vi "Query_source_settings_menu.vi"(8 "error in (no error)":errorcluster) -> (0 "error out":errorcluster, 1 "Cancelled?":bool, 3 "Output cluster":T1={"Integer Timestamp"=0, "Einzel Voltage"=0.0, "Needle Voltage"=0.0, "Frequency"=1.0, "Width (ms) : 0.1 "=0.05, "Desired Amplitude (V)"=0.0, "X Voltage"=0.0, "Y Voltage"=0.0, "Settings ID"="", "ID#"=0} {"Needle Voltage" min=0.0 max=10.0 step=0.01 format="%.2g"; "Y Voltage" min=0.0 max=9.0 step=0.01 format="%.2g"; "X Voltage" min=0.0 max=9.0 step=0.01 format="%.2g"; "Einzel Voltage" min=0.0 max=10.0 step=0.01 format="%.2g"; "Desired Amplitude (V)" min=0.0 max=10.0 step=0.01 format="%5.2f"; "Width (ms) : 0.1" min=0.05 max=5.0 step=0.01 format="%6.2f"; "Frequency" min=1.0 max=100.0 step=0.01 format="%.1f"})   [LabVIEW 2013]
doc: "Displays a standard dialog box that prompts users to enter information, such as a user name and password.\n--------------------\n\nThis Express VI is configured as follows:\n\nMessage to Display to the User:\nThe inputs are: \nNumber: Upper Timestamp Range\nNumber: Lower Timestamp Range\nNumber: Settings ID"
uses:
  Controls/dust_soruce_control.ctl
  Controls/Source_settings_select.ctl
  <vilib>/Utility/miscctls.llb/LVPointTypeDef.ctl
panel:
  out "Source Control Array":T1[](array[typedef]) {"Needle Voltage" min=0.0 max=10.0 step=0.01 format="%.2g"; "Y Voltage" min=0.0 max=9.0 step=0.01 format="%.2g"; "X Voltage" min=0.0 max=9.0 step=0.01 format="%.2g"; "Einzel Voltage" min=0.0 max=10.0 step=0.01 format="%.2g"; "Desired Amplitude (V)" min=0.0 max=10.0 step=0.01 format="%5.2f"; "Width (ms) : 0.1" min=0.05 max=5.0 step=0.01 format="%6.2f"; "Frequency" min=1.0 max=100.0 step=0.01 format="%.1f"}
  in  "Settings Type":T2
  in  "Clear Filter":bool
  in  "Tag Filter":T3
  in  "Load Settings":bool caption="OK2"
  in  "Cancel":bool
  in  "Settings ID":i32(ring) items=["Awesome settings that work"=30, "Awesome settings that work"=31, "Working settings"=35, "Working settings"=36, "Working settings"=37, "Working settings"=38, "Working settings"=39, ""=42, "Test"=43, "Test"=44, "Test"=46, "Test 1"=47, "Test 1"=48, "Anna's Settings"=49, "test of width"=51, "Anna's Settings (Updated with working Giraffes)"=72, "Anna's Settings (Updated with working Giraffes)"=73, "test"=75, "test"=76, "test 1"=77, "test 1"=78, "test 3"=82, "test 4"=83, "Anna's Settings"=86, "Anna's Settings1"=87, "test mctesty"=88, "test mctesty"=89, "Test\""=91, "Test\""=92, "this is a \"test\" setting"=93, "Test 'Test' \"Test\" test test."=97, "testsaved at  10/25/2012 3:26:30 PM"=101, "test (saved at  10/25/2012 3:26:53 PM)"=103, "Leela (saved at  11/2/2012 10:29:09 AM)"=112, "Light flash run 2 (saved at  11/13/2012 12:55:50 PM)"=184, "AnnaWorking (saved at  11/19/2012 12:04:04 PM)"=198, "AnnaWorking (saved at  11/19/2012 2:06:00 PM)"=200, "AnnaWorking (saved at  11/19/2012 4:00:30 PM)"=201, "DCS testing 1 (saved at  12/10/2012 3:10:12 PM)"=237, " (saved at  12/10/2012 6:22:18 PM)"=241, " (saved at  12/13/2012 1:54:08 PM)"=258, " (saved at  12/18/2012 1:57:42 PM)"=267, " (saved at  12/18/2012 1:57:45 PM)"=268, " (saved at  12/18/2012 1:58:11 PM)"=269, "fibera (saved at  12/18/2012 1:58:19 PM)"=270, "fibera (saved at  12/18/2012 1:58:37 PM)"=271, "fibera (saved at  12/18/2012 4:18:34 PM)"=272, "fibera (saved at  12/21/2012 11:52:02 AM)"=277, "Evan (saved at  2/11/2013 11:10:44 AM)"=346, "Evan (saved at  2/11/2013 11:10:45 AM)"=347, "Evan (saved at  2/11/2013 11:10:47 AM)"=348, "Evan (saved at  2/11/2013 11:10:48 AM)"=349, "Evan (saved at  2/11/2013 11:10:48 AM)"=350, "Evan (saved at  2/11/2013 11:10:48 AM)"=351, "Evan (saved at  2/11/2013 11:10:48 AM)"=352, "Evan (saved at  2/11/2013 11:10:48 AM)"=353, "Evan (saved at  2/11/2013 11:10:49 AM)"=354, "Evan (saved at  2/11/2013 11:10:50 AM)"=355, "Evan (saved at  2/11/2013 11:10:50 AM)"=356, "MINE (saved at  2/14/2013 11:07:05 AM)"=365, "MINE (saved at  2/14/2013 11:07:30 AM)"=366, "this (saved at  2/14/2013 12:24:07 PM)"=367, "this (saved at  2/14/2013 12:24:20 PM)"=368, "this (saved at  2/14/2013 12:24:20 PM)"=369, "this (saved at  2/14/2013 12:24:20 PM)"=370, "this (saved at  2/14/2013 12:24:21 PM)"=371, "this (saved at  2/14/2013 12:24:21 PM)"=372, "this (saved at  2/14/2013 12:24:21 PM)"=373, "MINE (saved at  2/14/2013 3:45:56 PM)"=374, " (saved at  2/18/2013 2:58:35 PM)"=379, "Evan (saved at  2/18/2013 2:58:43 PM)"=380, " (saved at  2/18/2013 5:00:50 PM)"=389, " (saved at  2/19/2013 11:55:54 AM)"=391, "Evan (saved at  2/19/2013 11:56:13 AM)"=392, "YABBADABBADOO (saved at  3/1/2013 10:24:08 AM)"=415, "Best Settings (saved at  5/6/2013 4:16:23 PM)"=473, "Aiming (saved at  5/21/2013 11:06:06 AM)"=548, "EVAN USE THESE SETTINGS (Freq: 15-20 ish) (saved at  5/21/2013 3:57:32 PM)"=552, "EVAN USE THESE SETTINGS (Freq: 15-20 ish) (saved at  5/21/2013 3:57:43 PM)"=553, "stereo (saved at  5/28/2013 12:22:49 PM)"=567, "stereo (saved at  5/28/2013 12:23:26 PM)"=568, "stereo (saved at  5/28/2013 1:04:18 PM)"=569, "stereo (saved at  5/28/2013 1:33:34 PM)"=570, "stereo (saved at  5/28/2013 1:33:38 PM)"=571, "test (saved at  5/31/2013 9:30:39 AM)"=573, "stereo (saved at  6/5/2013 4:20:29 PM)"=585, "stereo (saved at  6/11/2013 11:18:15 AM)"=590, "stereo (saved at  6/18/2013 5:04:42 PM)"=596, "stereo (saved at  6/20/2013 2:33:58 PM)"=600, "stereo (saved at  6/28/2013 10:16:59 AM)"=607, "stereo (saved at  7/16/2013 1:47:31 PM)"=611, "stereo (saved at  8/20/2013 5:15:00 PM)"=630, "stereo high (saved at  8/21/2013 11:26:34 AM)"=632, "stereo high (saved at  8/21/2013 2:57:56 PM)"=634, "stereo high focus better? (saved at  8/21/2013 4:20:43 PM)"=635, "stereo high focus better? (saved at  8/21/2013 4:22:36 PM)"=636, "aiming (saved at  8/27/2013 9:46:16 AM)"=640, "eric initial highspeed (saved at  8/29/2013 9:32:19 AM)"=641, "eric highspeed (saved at  8/29/2013 10:11:17 AM)"=642, "eric high S1 (saved at  8/29/2013 12:56:28 PM)"=643, "eric  S3 (saved at  8/29/2013 1:27:03 PM)"=645, "Solar Cell (saved at  9/17/2013 11:09:09 AM)"=656, "Solar Cell (saved at  9/17/2013 1:21:46 PM)"=657, "trytomakeolivineGO (saved at  9/23/2013 2:27:29 PM)"=664, "trytomakeolivineGO (saved at  9/23/2013 2:46:08 PM)"=666, "trytomakeolivineGO (saved at  9/23/2013 3:18:03 PM)"=667, "trytomakeolivineGO (saved at  9/23/2013 5:08:18 PM)"=669, "trytomakeolivineGO (saved at  9/24/2013 9:55:57 AM)"=673, "olivinehigh (saved at  9/24/2013 5:17:27 PM)"=679, "olivineisshooting (saved at  9/25/2013 10:27:24 AM)"=682, "olivineisshooting (saved at  9/25/2013 10:28:24 AM)"=683, "olivineisshooting? (saved at  9/25/2013 2:02:32 PM)"=684, "reallyhigh (saved at  9/26/2013 2:34:23 PM)"=690, "OLIVINE (saved at  9/30/2013 9:57:31 AM)"=693, "OLIVINE (saved at  9/30/2013 11:18:54 AM)"=694, "OLIVINE (saved at  9/30/2013 5:13:02 PM)"=696, "OLIVINE (saved at  10/2/2013 10:01:39 AM)"=699, "OLIVINE (saved at  10/2/2013 2:01:51 PM)"=701, "OLIVINE 1MV (saved at  10/2/2013 3:00:49 PM)"=703, "OLIVINE (saved at  10/3/2013 1:12:46 PM)"=705, "OLIVINE (saved at  10/3/2013 2:06:14 PM)"=709, "OLIVINE (saved at  10/3/2013 2:55:49 PM)"=711, "OLIVINE (saved at  10/3/2013 3:10:16 PM)"=712, "OLIVINE (saved at  10/3/2013 5:08:59 PM)"=714, "OLIVINE (saved at  10/4/2013 10:04:38 AM)"=716, "OLIVINE (saved at  10/4/2013 10:38:50 AM)"=718, "starting slow (saved at  10/9/2013 11:50:46 AM)"=721, "starting slow (saved at  10/9/2013 1:21:22 PM)"=723, "starting slow (saved at  10/9/2013 1:50:43 PM)"=725, "starting slow (saved at  10/9/2013 1:56:23 PM)"=727, "starting slow (saved at  10/9/2013 4:04:05 PM)"=729, "starting slow (saved at  10/9/2013 4:45:52 PM)"=731, "starting slow (saved at  10/9/2013 4:45:57 PM)"=732, "starting slow (saved at  10/9/2013 5:19:49 PM)"=733, "Throop Foils (saved at  10/14/2013 10:53:03 AM)"=735, "Throop Foils (saved at  10/16/2013 4:10:58 PM)"=736, "Throop Foils (saved at  10/16/2013 4:27:11 PM)"=737, "stereo (saved at  10/21/2013 11:06:33 AM)"=738, "stereo (saved at  10/24/2013 10:50:29 AM)"=743, "stereo (saved at  10/25/2013 3:04:38 PM)"=745, "stereo (saved at  10/25/2013 3:24:02 PM)"=746, "stereo (saved at  10/31/2013 3:12:55 PM)"=750, "stereo (saved at  11/6/2013 9:02:15 AM)"=752, "2013_1111_best (saved at  11/11/2013 6:07:39 PM)"=755, "2013_1112_best (saved at  11/12/2013 9:31:19 AM)"=756, "2013_1112_best (saved at  11/12/2013 3:37:27 PM)"=757, "Best_NDA (saved at  11/27/2013 11:44:34 AM)"=758, "Best_NDA (saved at  12/5/2013 11:49:56 AM)"=789, "Graphite-2-1 (saved at  1/13/2014 9:22:39 AM)"=814, "Graphite-2-1 (saved at  1/13/2014 9:49:16 AM)"=817, "Graphite-2-1 (saved at  1/14/2014 10:59:32 AM)"=875, "2014_01_20_olivine (saved at  1/20/2014 12:33:33 PM)"=944, "olivine_ldex (saved at  1/21/2014 10:41:30 AM)"=949, "olivine_ldex 5-10 (saved at  1/24/2014 12:04:35 PM)"=977, "LDEX: olivine (saved at  1/30/2014 12:36:57 PM)"=1020, "LDEX: olivine slow (saved at  2/3/2014 10:46:14 AM)"=1032, "LDEX olivine callibration (saved at  2/4/2014 4:17:00 PM)"=1064, "LDEX olivine callibration (saved at  2/5/2014 8:47:13 AM)"=1071, "LDEX olivine callibration 2.2 (saved at  2/5/2014 8:57:15 AM)"=1073, "LDEX olivine callibration 1.8 (saved at  2/5/2014 9:34:21 AM)"=1077, "LDEX olivine callibration 1.6 (saved at  2/5/2014 10:15:07 AM)"=1081, "slow speeds (DT: Iron-3-2; HV: 2.2;  time: 2/17/2014 9:43:43 AM)"=1172, "bes (DT: Iron-3-2; HV: 2.2;  time: 2/17/2014 3:46:29 PM)"=1210, "best (DT: Iron-3-2; HV: 2.2;  time: 2/19/2014 9:24:22 AM)"=1234, "best (DT: Iron-3-2; HV: 2.2;  time: 3/11/2014 1:52:00 PM)"=1329, "ODINSun (DT: Iron-3-2; HV: 2.2;  time: 4/17/2014 4:19:54 PM)"=1477, "Best Settings (DT: Mix-3-1; HV: 2.2;  time: 4/22/2014 9:50:01 AM)"=1489, " (DT: Mix-3-1; HV: 2.7;  time: 5/13/2014 2:53:24 PM)"=1598, " (DT: Mix-5-1; HV: 2.2;  time: 5/28/2014 4:29:56 PM)"=1612, "MM1 Iron 5-1 (DT: Mix-5-1; HV: 2.2;  time: 5/28/2014 4:30:58 PM)"=1613, "MM1 Lifetest Iron 5-1 (DT: Mix-5-1; HV: 2.2;  time: 5/28/2014 4:46:22 PM)"=1615, "MM1 Lifetest Iron 5-1 (DT: Mix-5-1; HV: 2.2;  time: 5/29/2014 5:22:11 PM)"=1642, "MM1 Lifetest Iron 5-1 (Left alone) (DT: Mix-5-1; HV: 2.2;  time: 6/2/2014 8:40:21 PM)"=1769, "best nickel (DT: Nickel-1-1; HV: 2.2;  time: 6/17/2014 10:17:39 AM)"=1812, " (DT: Nickel-1-1; HV: 2.2;  time: 6/27/2014 12:46:40 PM)"=1865, "July 1, Good Nickel (DT: Nickel-1-1; HV: 2.2;  time: 7/1/2014 12:38:28 PM)"=1876, "30hz to start (DT: Nickel-1-1; HV: 2.2;  time: 7/4/2014 12:55:47 PM)"=1898, "Running okay (DT: Iron-1E+1-1; HV: 2.2;  time: 8/19/2014 9:04:38 AM)"=1957, "DCSI (DT: Iron-1E+1-1; HV: 2.2;  time: 9/2/2014 1:54:57 PM)"=2004, "Eric Christian >25km/s particles (DT: Iron-1E+1-1; HV: 2.2;  time: 10/8/2014 12:51:10 PM)"=2111, "Eric Christian >5-10km/s particles (DT: Iron-1E+1-1; HV: 2.2;  time: 10/9/2014 1:01:25 PM)"=2136, "Starting Point (DT: Iron-1E+1-1; HV: 2.2;  time: 11/10/2014 1:22:02 PM)"=2278, "Iron Low Peletron Voltage First attempt (DT: Iron-1E+1-1; HV: 0.8;  time: 12/18/2014 6:17:52 PM)"=2999, "Iron Low Peletron Voltage a bit better (DT: Iron-1E+1-1; HV: 0.8;  time: 12/18/2014 6:36:23 PM)"=3003, "Iron Low Peletron Voltage.  Settings seem to be better for slow, small particles. (DT: Iron-1E+1-1; HV: 0.8;  time: 12/18/2014 7:03:42 PM)"=3009, "Iron Low Peletron Voltage.  Settings seem to be better for slow, small particles. (DT: Iron-1E+1-1; HV: 2.2;  time: 1/8/2015 12:14:42 PM)"=3038, "Georg STEREO settings (DT: Iron-1E+1-1; HV: 2.2;  time: 1/8/2015 12:14:57 PM)"=3039, "best (DT: Iron-1E+1-1; HV: 2.2;  time: 2/11/2015 12:24:40 PM)"=3236, "best >10 (DT: Iron-1E+1-1; HV: 2.2;  time: 2/11/2015 12:43:56 PM)"=3240, "Iron starting to shoot (DT: Iron-1E+1-1; HV: 2.2;  time: 2/15/2015 12:40:16 PM)"=3263, ">10 shooting (DT: Iron-1E+1-1; HV: 2.2;  time: 2/18/2015 11:04:22 AM)"=3292, " (DT: Iron-1E+1-1; HV: 1.2;  time: 4/20/2015 2:34:18 PM)"=3596, "STEREO CSA (DT: Iron-1E+1-2; HV: 2.2;  time: 7/20/2015 5:52:18 PM)"=3861, "STEREO CSA (DT: Iron-1E+1-2; HV: 2.2;  time: 7/20/2015 5:52:40 PM)"=3862]
  in  "Lower Timestamp Range":timestamp
  in  "Upper Timestamp Range":timestamp
  in  "Einzel Voltage":dbl
  in  "Needle Voltage":dbl
  in  "Frequency":dbl
  in  "Width (ms) : 0.1":dbl
  in  "Desired Amplitude (V)":dbl
  in  "X Voltage":dbl
  in  "Y Voltage":dbl
  out "Settings to be loaded":string
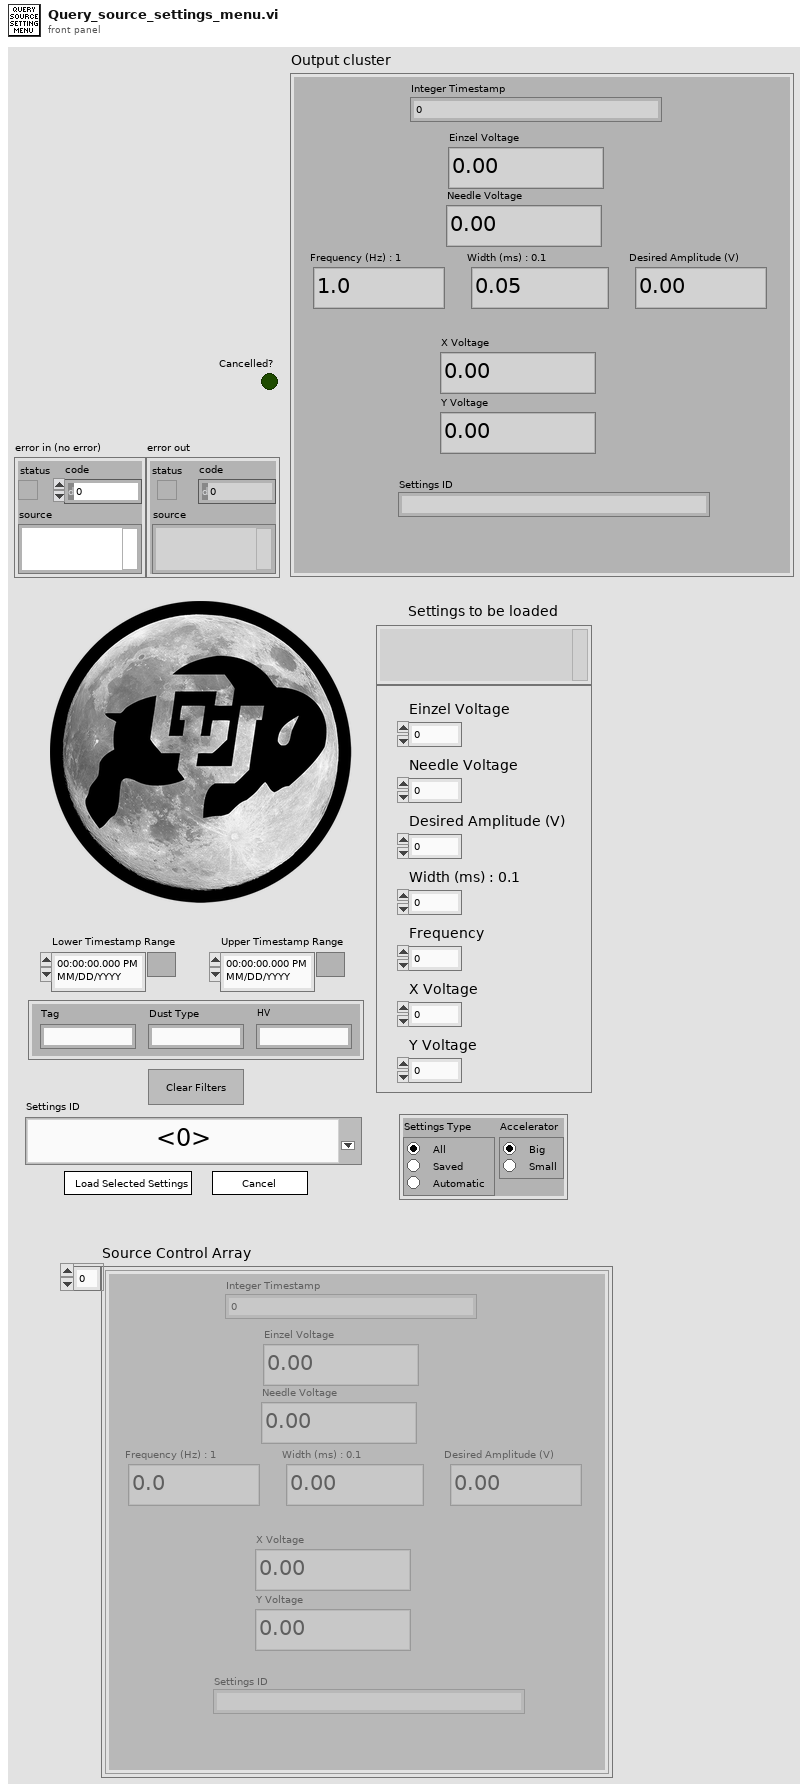
[diagram p1: front panel]
types:
  T1 = typedef "dust_soruce_control.ctl" = cluster{"Integer Timestamp":u64, "Einzel Voltage":dbl, "Needle Voltage":dbl, "Frequency":dbl, "Width (ms) : 0.1 ":dbl, "Desired Amplitude (V)":dbl, "X Voltage":dbl, "Y Voltage":dbl, "Settings ID":string, "ID#":i32}
  T2 = typedef "Source_settings_select.ctl" = cluster{"Settings Type":enum32{"All", "Saved", "Automatic"}, "Accelerator":enum32{"Big", "Small"}}
  T3 = cluster{"Tag":string, "Dust Type":string, "HV":string}
  T4 = typedef "LVPointTypeDef.ctl" = cluster{"Horizontal":i16, "Vertical":i16}
  T5 = enum8{"Enabled", "Disabled", "Disabled and Grayed Out"}
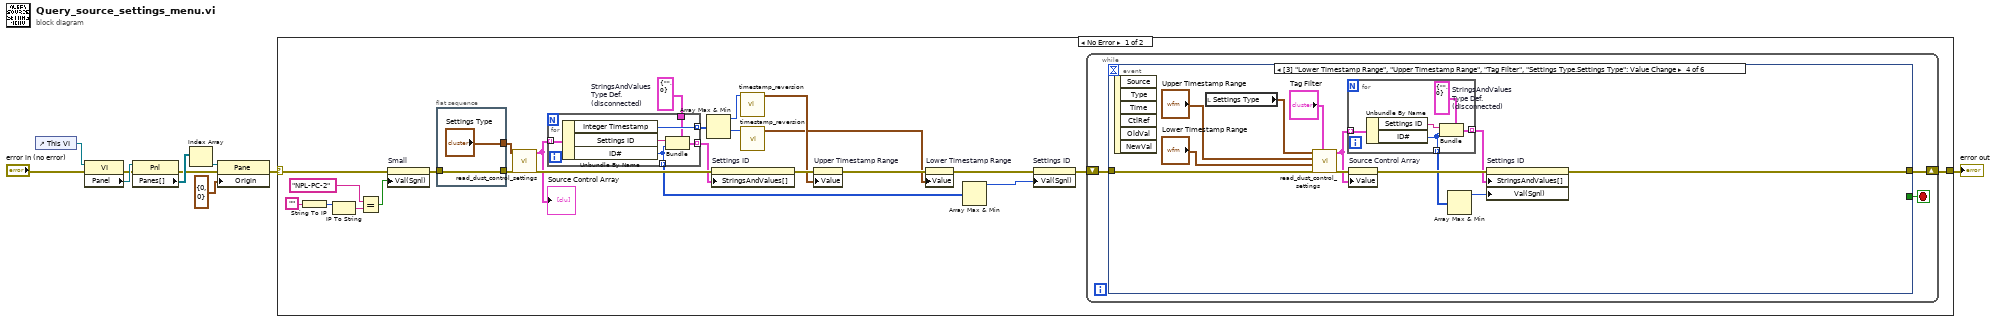
[diagram p0: block diagram]
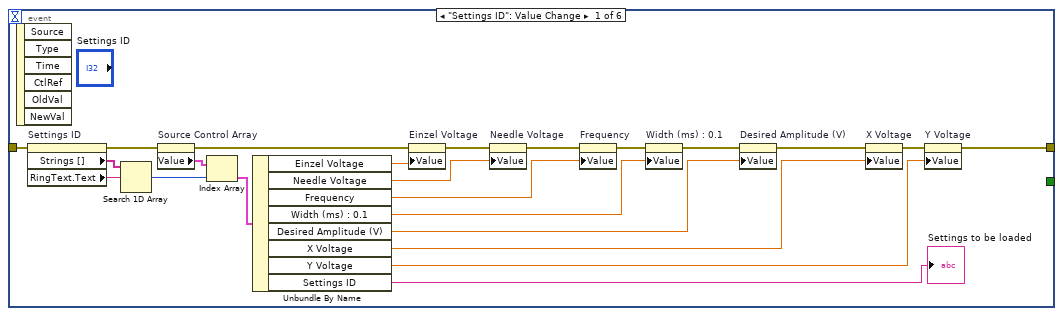
[diagram p2: hidden frame]
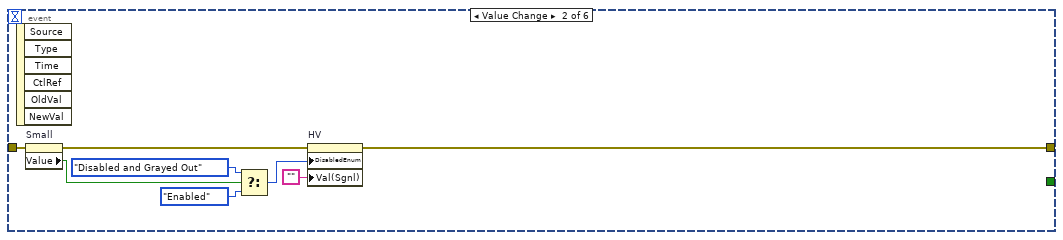
[diagram p3: hidden frame]
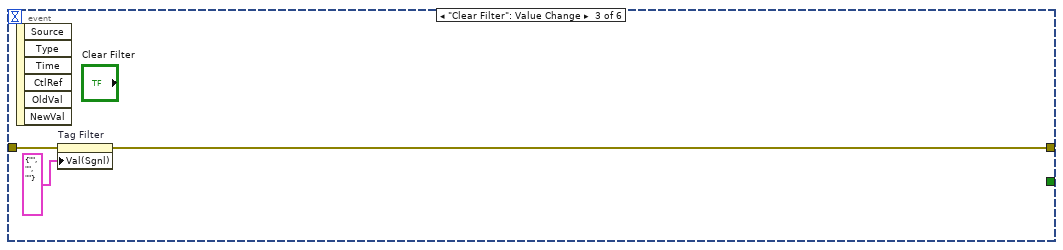
[diagram p4: hidden frame]
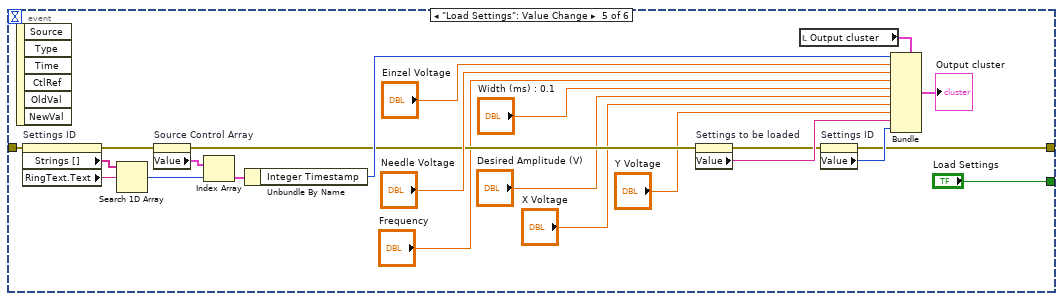
[diagram p5: hidden frame]
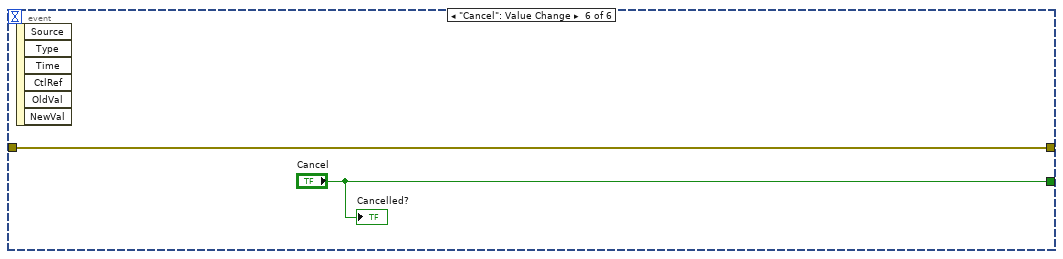
[diagram p6: hidden frame]
diagram:
  n1 = control-ref of="This VI"() -> (w3:refnum<vi>)
  n2 = property class="VI"(reference=w3, error in="error in (no error)") -> (error out=w4:errorcluster, "Panel"=w5:refnum<vi>)  [unwired: 1 out]
  n3 = property class="Pnl"(reference=w5, error in=w4) -> (error out=w6:errorcluster, "Panes[]"=w7:refnum<vi>[])  [unwired: 1 out]
  n4 = Index Array(array=w7) -> (element=w8:refnum<vi>)  [unwired: 1 in]
  n5 = property class="Pane"(reference=w8, error in=w6, "Origin"=T4 {"Horizontal"=0, "Vertical"=0}) -> (error out=w1:errorcluster)  [unwired: 1 out]
  n6 = case shown="No Error" w1 {
    selector: w1 -> [w11 w123]
    tunnel: [w19 w123] -> w10
    frame No Error {
      w33 = cluster{"String":string, "Value":i32} {"String"="", "Value"=0}  # StringsAndValues Type Def. (disconnected)
      n7 = String To IP(1:"") -> (0:w17:u32)
      n8 = IP To String(2:w17) -> (0:w16:string)  [unwired: 1 in]
      n9 = Equal?(x="NPL-PC-2", y=w16) -> (x = y?=w14:bool)
      n10 = property on="Small" class="Bool (strict)"(error in=w11, "Val(Sgnl)"=w14) -> (error out=w12:errorcluster)  [unwired: 1 in, 1 out]
      n11 = flat-sequence {
        tunnel: ["Settings Type"] -> w24
        tunnel: [w36] -> w13
        tunnel: w12 -> [w36]
        frame #0 {
        }
      }
      n12 = call "read_dust_control_settings.vi"("error in (no error)"=w13, "Settings Type"=w24) -> ("error out"=w34:errorcluster, "Source Control Array"=w25:T1[])  [unwired: 8 in]
      "Source Control Array" <- w25
      n13 = for {
        tunnel: w25 -> [w122] mode=indexing
        tunnel: [w121] -> w35 mode=indexing
        tunnel: w33 -> [w120]
        tunnel: [w118] -> w32 mode=indexing
        tunnel: [w117] -> w21 mode=indexing
        n14 = Unbundle By Name(w122) -> ("Integer Timestamp"=w121:u64, "Settings ID"=w119:string, "ID#"=w117:i32)
        n15 = Bundle(cluster=w120, "String"=w119, "Value"=w117) -> (w118:cluster{"String":string, "Value":i32})
      }
      n16 = Array Max & Min(array=w35) -> (max value=w31:u64, min value=w30:u64)  [unwired: 2 out]
      n17 = property on="Settings ID" class="Ring (strict)"(error in=w34, "StringsAndValues[]"=w32) -> (error out=w29:errorcluster)  [unwired: 1 in, 1 out]
      n18 = call "timestamp_reversion.vi"("Integer Timestamp"=w31) -> ("time stamp"=w28:timestamp)  [unwired: 8 in, 1 out]
      n19 = call "timestamp_reversion.vi"("Integer Timestamp"=w30) -> ("time stamp"=w26:timestamp)  [unwired: 8 in, 1 out]
      n20 = property on="Upper Timestamp Range" class="AbsTime (strict)"(error in=w29, "Value"=w28) -> (error out=w27:errorcluster)  [unwired: 1 in, 1 out]
      n21 = property on="Lower Timestamp Range" class="AbsTime (strict)"(error in=w27, "Value"=w26) -> (error out=w23:errorcluster)  [unwired: 1 in, 1 out]
      n22 = Array Max & Min(array=w21) -> (max value=w20:i32)  [unwired: 3 out]
      n23 = property on="Settings ID" class="Ring (strict)"(error in=w23, "Val(Sgnl)"=w20) -> (error out=w22:errorcluster)  [unwired: 1 in, 1 out]
      n24 = while {
        shift-right: [w40] -> w19
        shift-left: w22 -> [w39]
        stop <- w38 stop-if-true
        n25 = event shown="[3] \"Lower Timestamp Range\", \"Upper Timestamp Range\", \"Tag Filter\", \"Settings Type.Settings Type\": Value Change" {
          selector: _ -> [_ _ _ _ _ _]
          dyn-events: _ -> [_ _ _ _ _ _]
          timeout: _ -> [_ _ _ _ _ _]
          tunnel: [w42 w65 w72 w77 w111 w116] -> w40
          tunnel: w39 -> [w63 w71 w74 w86 w109 w116]
          tunnel: [_ _ _ _ "Load Settings" "Cancel"] -> w38
          event "Settings ID": Value Change {
            n26 = event-data() -> ()  [unwired: 1 in, 6 out]
            n27 = property on="Settings ID" class="Ring (strict)"(error in=w63) -> (error out=w58:errorcluster, "Strings []"=w59:string[], "RingText.Text"=w62:string)  [unwired: 1 in, 1 out]
            n28 = Search 1D Array(1D array=w59, element=w62) -> (index of element=w60:i32)  [unwired: 1 in]
            n29 = property on="Source Control Array" class="Arr (strict)"(error in=w58) -> (error out=w56:errorcluster, "Value"=w61:T1[])  [unwired: 1 in, 1 out]
            n30 = Index Array(array=w61, index=w60) -> (element=w57:T1)
            n31 = Unbundle By Name(w57) -> ("Einzel Voltage"=w55:dbl, "Needle Voltage"=w54:dbl, "Frequency"=w53:dbl, "Width (ms) : 0.1"=w52:dbl, "Desired Amplitude (V)"=w51:dbl, "X Voltage"=w50:dbl, "Y Voltage"=w49:dbl, "Settings ID"=→"Settings to be loaded":string)
            n32 = property on="Einzel Voltage" class="DigNum (strict)"(error in=w56, "Value"=w55) -> (error out=w48:errorcluster)  [unwired: 1 in, 1 out]
            n33 = property on="Needle Voltage" class="DigNum (strict)"(error in=w48, "Value"=w54) -> (error out=w47:errorcluster)  [unwired: 1 in, 1 out]
            n34 = property on="Frequency" class="DigNum (strict)"(error in=w47, "Value"=w53) -> (error out=w46:errorcluster)  [unwired: 1 in, 1 out]
            n35 = property on="Width (ms) : 0.1" class="DigNum (strict)"(error in=w46, "Value"=w52) -> (error out=w45:errorcluster)  [unwired: 1 in, 1 out]
            n36 = property on="Desired Amplitude (V)" class="DigNum (strict)"(error in=w45, "Value"=w51) -> (error out=w44:errorcluster)  [unwired: 1 in, 1 out]
            n37 = property on="X Voltage" class="DigNum (strict)"(error in=w44, "Value"=w50) -> (error out=w43:errorcluster)  [unwired: 1 in, 1 out]
            n38 = property on="Y Voltage" class="DigNum (strict)"(error in=w43, "Value"=w49) -> (error out=w42:errorcluster)  [unwired: 1 in, 1 out]
          }
          event Value Change {
            n39 = event-data() -> ()  [unwired: 1 in, 6 out]
            n40 = property on="Small" class="Bool (strict)"(error in=w71) -> (error out=w70:errorcluster, "Value"=w66:bool)  [unwired: 1 in, 1 out]
            n41 = Select(t=T5."Disabled and Grayed Out" ("Disabled"), s=w66, f=T5."Enabled" ("Disabled")) -> (s? t:f=w68:T5)
            n42 = property on="HV" class="Str"(error in=w70, "DisabledEnum"=w68, "Val(Sgnl)"="" ("Value (Signaling)")) -> (error out=w65:errorcluster)  [unwired: 1 in, 1 out]
          }
          event "Clear Filter": Value Change {
            n43 = event-data() -> ()  [unwired: 1 in, 6 out]
            n44 = property on="Tag Filter" class="Clust (strict)"(error in=w74, "Val(Sgnl)"=T3 {"Tag"="", "Dust Type"="", "HV"=""} ("Value (Signaling)")) -> (error out=w72:errorcluster)  [unwired: 1 in, 1 out]
          }
          event "Lower Timestamp Range", "Upper Timestamp Range", "Tag Filter": Value Change {
            n45 = event-data() -> ()  [unwired: 1 in, 6 out]
            n46 = local read "Settings Type"() -> (w85:T2)
            n47 = call "read_dust_control_settings.vi"("Query Cluster"="Tag Filter", "error in (no error)"=w86, "Lower Timestamp Range"="Lower Timestamp Range", "Upper Timestamp Range"="Upper Timestamp Range", "Settings Type"=w85) -> ("error out"=w81:errorcluster, "Source Control Array"=w80:T1[])  [unwired: 5 in]
            n48 = for {
              tunnel: w80 -> [w91] mode=indexing
              tunnel: [w88] -> w78 mode=indexing
              tunnel: [w87] -> w76 mode=indexing
              w89 = cluster{"String":string, "Value":i32} {"String"="", "Value"=0}  # StringsAndValues Type Def. (disconnected)
              n49 = Unbundle By Name(w91) -> ("Settings ID"=w90:string, "ID#"=w87:i32)
              n50 = Bundle(cluster=w89, "String"=w90, "Value"=w87) -> (w88:cluster{"String":string, "Value":i32})
            }
            n51 = property on="Source Control Array" class="Arr (strict)"(error in=w81, "Value"=w80) -> (error out=w79:errorcluster)  [unwired: 1 in, 1 out]
            n52 = Array Max & Min(array=w76) -> (max value=w75:i32)  [unwired: 3 out]
            n53 = property on="Settings ID" class="Ring (strict)"(error in=w79, "StringsAndValues[]"=w78, "Val(Sgnl)"=w75) -> (error out=w77:errorcluster)  [unwired: 1 in, 1 out]
          }
          event "Load Settings": Value Change {
            n54 = event-data() -> ()  [unwired: 1 in, 6 out]
            n55 = property on="Settings ID" class="Ring (strict)"(error in=w109) -> (error out=w106:errorcluster, "Strings []"=w108:string[], "RingText.Text"=w107:string)  [unwired: 1 in, 1 out]
            n56 = Search 1D Array(1D array=w108, element=w107) -> (index of element=w105:i32)  [unwired: 1 in]
            n57 = property on="Source Control Array" class="Arr (strict)"(error in=w106) -> (error out=w97:errorcluster, "Value"=w104:T1[])  [unwired: 1 in, 1 out]
            n58 = Index Array(array=w104, index=w105) -> (element=w103:T1)
            n59 = Unbundle By Name(w103) -> ("Integer Timestamp"=w102:u64)
            n60 = property on="Settings to be loaded" class="Str"(error in=w97) -> (error out=w100:errorcluster, "Value"=w101:string)  [unwired: 1 in, 1 out]
            n61 = local read "Output cluster"() -> (w113:T1)
            n62 = property on="Settings ID" class="Ring (strict)"(error in=w100) -> (error out=w111:errorcluster, "Value"=w112:i32)  [unwired: 1 in, 1 out]
            n63 = Bundle(cluster=w113, "Integer Timestamp"=w102, "Einzel Voltage"="Einzel Voltage", "Needle Voltage"="Needle Voltage", "Frequency"="Frequency", "Width (ms) : 0.1"="Width (ms) : 0.1", "Desired Amplitude (V)"="Desired Amplitude (V)", "X Voltage"="X Voltage", "Y Voltage"="Y Voltage", "Settings ID"=w101, "ID#"=w112) -> (→"Output cluster":T1)
          }
          event "Cancel": Value Change {
            n64 = event-data() -> ()  [unwired: 1 in, 6 out]
            "Cancelled?" <- "Cancel"
          }
        }
      }
    }
    frame Error {
    }
  }
  "error out" <- w10
